vi "Read Disabled.vi"(8 "error in (no error)":errorcluster, 11 "Disabled Assertion in":refnum<class "Disabled Assertion.lvclass">) -> (0 "error out":errorcluster, 2 "Disabled":T1(ring), 3 "Disabled Assertion out":refnum<class "Disabled Assertion.lvclass">)   [LabVIEW 2020, in "MacroAssert.lvlib" / "Disabled Assertion.lvclass"]
uses:
  Disabled Assertion.lvclass
  Disabled Assertion.lvclass/Disabled Assertion.ctl
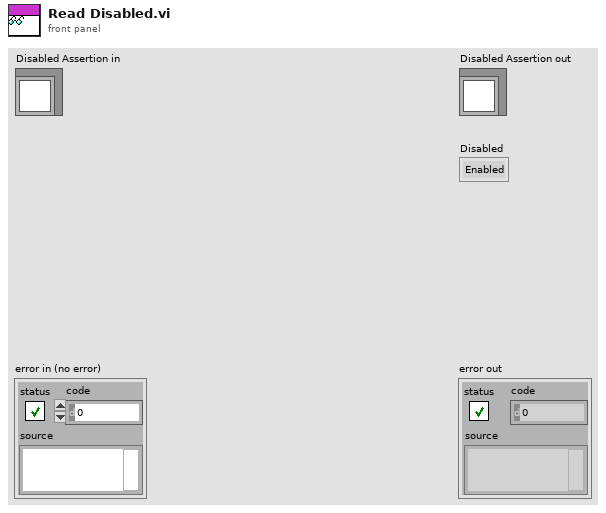
[diagram p1: front panel]
types:
  T1 = enum8{"Enabled", "Disabled", "Disabled and Grayed Out"}
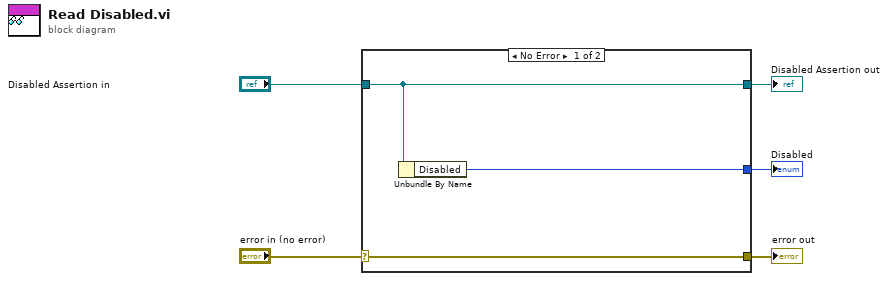
[diagram p0: block diagram]
diagram:
  n1 = case shown="No Error" "error in (no error)" {
    selector: "error in (no error)" -> [w8 w9]
    tunnel: [w8 w9] -> w4
    tunnel: [w7 w10] -> w2
    tunnel: "Disabled Assertion in" -> [w7 w10]
    tunnel: [w6 _] -> w1
    frame No Error {
      n2 = Unbundle By Name(w7) -> ("Disabled"=w6:T1)
    }
    frame Error {
    }
  }
  "error out" <- w4
  "Disabled Assertion out" <- w2
  "Disabled" <- w1
